vi "ReverseDir.vi"(1 "Direction":T1) -> (0 "Direction Out":T1)   [LabVIEW 2017, in "Atom.lvclass"]
uses:
  Atom.lvclass
  Type Defs/Direction Enum.ctl
  Type Defs/SB Type Defs.lvlib
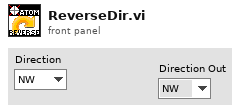
[diagram p1: front panel]
types:
  T1 = typedef "SB Type Defs.lvlib/Direction Enum.ctl" = enum16{"NW", "N", "NE", "E", "SE", "S", "SW", "W"}
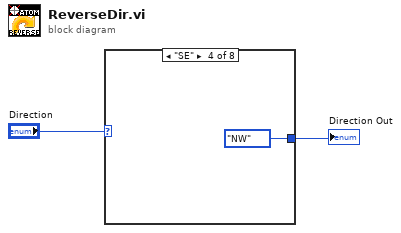
[diagram p0: block diagram]
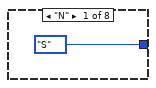
[diagram p2: hidden frame]
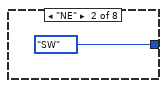
[diagram p3: hidden frame]
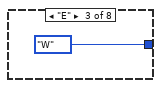
[diagram p4: hidden frame]
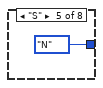
[diagram p5: hidden frame]
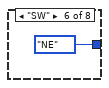
[diagram p6: hidden frame]
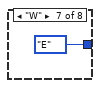
[diagram p7: hidden frame]
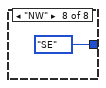
[diagram p8: hidden frame]
diagram:
  n1 = case shown="\"SE\"" "Direction" {
    tunnel: [Direction_Enum."S" ("Direction Out") Direction_Enum."SW" ("Direction Out") Direction_Enum."W" ("Direction Out") Direction_Enum."NW" ("Direction Out") Direction_Enum."N" ("Direction Out") Direction_Enum."NE" ("Direction Out") Direction_Enum."E" ("Direction Out") Direction_Enum."SE" ("Direction Out")] -> w1
    frame "N" {
    }
    frame "NE" {
    }
    frame "E" {
    }
    frame "SE" {
    }
    frame "S" {
    }
    frame "SW" {
    }
    frame "W" {
    }
    frame "NW" {
    }
  }
  "Direction Out" <- w1
